vi "Photon Counter Start.vi"(8 "errorIN":errorcluster caption="Error In", 11 "VISA resource name":refnum<visa-resource-name>) -> (0 "errorOUT":errorcluster caption="Error Out", 3 "VISA resource name out":refnum<visa-resource-name>)   [LabVIEW 2011, in "SR400.lvlib"]
uses:
  <instrlib>/SR400/SR400.lvlib
  <instrlib>/SR400/Public/Typedefs/Counter.ctl
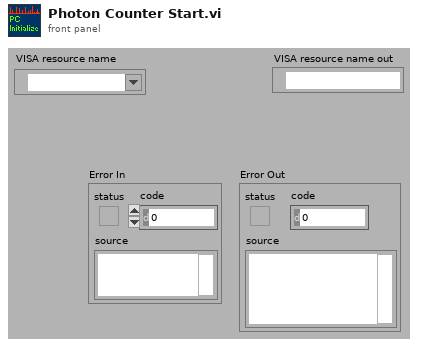
[diagram p1: front panel]
types:
  T1 = typedef "SR400.lvlib/Counter.ctl" = enum16{"Counter A", "Counter B", "Counter T"}
  T2 = enum16{"A,B For T Preset", "A-B For T Preset", "A+B For T Preset", "A For B Preset"}
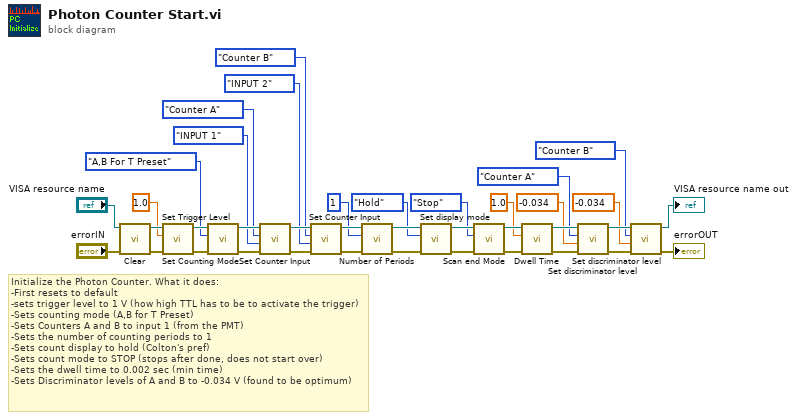
[diagram p0: block diagram]
diagram:
  # "Initialize the Photon Counter. What it does:\n-First resets to default\n-sets trigger level to 1 V (how high TTL has to be to activate the trigger) \n-Sets counting mode (A,B for T Preset)\n-Sets Counters A and B to input 1 (from the PMT)\n-Sets the number of counting periods to 1\n-Sets count display to hold (Colton's pref)\n-Sets count mode to STOP (stops after done, does not start over)\n-Sets the dwell time to 0.002 sec (min time)\n-Sets Discriminator levels of A and B to -0.034 V (found to be optimum)"
  n1 = call <instrlib>:"Clear.vi"("error in (no error)"="errorIN", "VISA resource name"="VISA resource name") -> ("error out"=w37:errorcluster, "VISA resource name out"=w38:refnum<visa-resource-name>)  [unwired: 8 out]
  n2 = call <instrlib>:"Set Trigger Level.vi"("error in (no error)"=w37, "Trigger Level (1 V)"=1.0 ("v (0.000000)"), "VISA resource name"=w38) -> ("error out"=w35:errorcluster, "VISA resource name out"=w36:refnum<visa-resource-name>)  [unwired: 7 out]
  n3 = call <instrlib>:"Set Counting Mode.vi"("error in (no error)"=w35, "Mode (def: A,B for T preset)"=T2."A,B For T Preset" ("i (0) 2"), "VISA resource name"=w36) -> ("error out"=w33:errorcluster, "VISA resource name out"=w34:refnum<visa-resource-name>)  [unwired: 7 out]
  n4 = call <instrlib>:"Set Counter Input.vi"("error in (no error)"=w33, "Input (def: 10 MHz)"=enum16{"10 MHz", "INPUT 1", "INPUT 2", "TRIG"}."INPUT 1" ("n (0.000000)"), "Counter (def: A)"=enum16{"Counter A", "Counter B", "Counter T"}."Counter A" ("i (0) 2"), "VISA resource name"=w34) -> ("error out"=w31:errorcluster, "VISA resource name out"=w32:refnum<visa-resource-name>)  [unwired: 6 out]
  n5 = call <instrlib>:"Set Counter Input.vi"("error in (no error)"=w31, "Input (def: 10 MHz)"=enum16{"10 MHz", "INPUT 1", "INPUT 2", "TRIG"}."INPUT 2" ("n (0.000000)"), "Counter (def: A)"=enum16{"Counter A", "Counter B", "Counter T"}."Counter B" ("i (0) 2"), "VISA resource name"=w32) -> ("error out"=w19:errorcluster, "VISA resource name out"=w20:refnum<visa-resource-name>)  [unwired: 6 out]
  n6 = call <instrlib>:"Number of Periods.vi"("error in (no error)"=w19, "# of periods (def: 1)"=1 ("m (1)"), "VISA resource name"=w20) -> ("error out"=w29:errorcluster, "VISA resource name out"=w30:refnum<visa-resource-name>)  [unwired: 7 out]
  n7 = call <instrlib>:"Set display mode.vi"("error in (no error)"=w29, "Display Mode (def: Hold)"=enum16{"Continuous", "Hold"}."Hold", "VISA resource name"=w30) -> ("error out"=w27:errorcluster, "VISA resource name out"=w28:refnum<visa-resource-name>)  [unwired: 7 out]
  n8 = call <instrlib>:"Scan end Mode.vi"("error in (no error)"=w27, "Scan End Mode (Def: Stop)"=enum16{"Stop", "Start"}."Stop", "VISA resource name"=w28) -> ("error out"=w25:errorcluster, "VISA resource name out"=w26:refnum<visa-resource-name>)  [unwired: 7 out]
  n9 = call "Dwell Time.vi"("error in (no error)"=w25, "Dwell time (0.002 s)"=1.0 ("x (0.000000)"), "VISA resource name"=w26) -> ("error out"=w23:errorcluster, "VISA resource name out"=w24:refnum<visa-resource-name>)  [unwired: 7 out]
  n10 = call <instrlib>:"Set discriminator level.vi"("error in (no error)"=w23, "Level (-0.034 V)"=-0.034 ("v (0.000000)"), "Discriminator (def: A)"=Counter."Counter A", "VISA resource name"=w24) -> ("error out"=w21:errorcluster, "VISA resource name out"=w22:refnum<visa-resource-name>)  [unwired: 6 out]
  n11 = call <instrlib>:"Set discriminator level.vi"("error in (no error)"=w21, "Level (-0.034 V)"=-0.034 ("v (0.000000)"), "Discriminator (def: A)"=Counter."Counter B", "VISA resource name"=w22) -> ("error out"=→"errorOUT":errorcluster, "VISA resource name out"=→"VISA resource name out":refnum<visa-resource-name>)  [unwired: 6 out]
